vi "datataker_binary.vi"() -> ()   [LabVIEW 2012]
doc: "This example demonstrates how to acquire a single buffer of voltage measurements using a DAQmx device.\n\nFor instructions on how to connect your signals to the DAQ device, refer to your device documentation."
uses:
  <vilib>/userdefined/High Color/nirio_resource_hc.ctl
  <vilib>/Utility/error.llb/DialogType.ctl
  <vilib>/addons/h5labview2/file/H5Fmode.ctl
  <vilib>/DAQmx/write.llb/DAQmx Write (Analog 1D DBL 1Chan NSamp).vi
  <vilib>/DAQmx/read.llb/DAQmx Read (Analog 2D DBL NChan NSamp).vi
  <vilib>/addons/h5labview2/base/lib_path.vi
  <vilib>/DAQmx/read.llb/DAQmx Read (Analog 1D Wfm NChan NSamp).vi
  <vilib>/FPGAPlugInAG/PCIe-7841R/niLvFpga_Open_PCIe-7841R.vi
  <vilib>/DAQmx/create/channels.llb/DAQmx Create Channel (AI-Voltage-Basic).vi
  <vilib>/DAQmx/configure/timing.llb/DAQmx Timing (Sample Clock).vi
  <vilib>/DAQmx/configure/task.llb/DAQmx Configure Logging (TDMS).vi
  <vilib>/DAQmx/configure/trigger.llb/DAQmx Start Trigger (Digital Edge).vi
  <vilib>/DAQmx/configure/trigger.llb/DAQmx Start Trigger (Analog Edge).vi
  <vilib>/DAQmx/configure/trigger.llb/DAQmx Reference Trigger (Digital Edge).vi
  <vilib>/DAQmx/configure/trigger.llb/DAQmx Reference Trigger (Analog Edge).vi
  <vilib>/Utility/error.llb/Error Cluster From Error Code.vi
  <vilib>/rvi/errors/niLvFpgaAdjustHostInterfaceError.vi
  <vilib>/DAQmx/miscellaneous.llb/DAQmx Fill In Error Info.vi
  <vilib>/addons/h5labview2/base/H5Equery.vi
  Multiple Waveforms.vi
  <vilib>/Waveform/WDTFileIO.llb/Export Waveforms To Spreadsheet File (1D).vi
  <vilib>/DAQmx/create/channels.llb/DAQmx Create Channel (AO-Voltage-Basic).vi
  <vilib>/rvi/interface/nirviOpenFPGA/nirviOpenFPGA.xnode
  fpga/MultiChannelFeed_FPGATarget2_feedbackcooling(_T5hmXv3JUos.lvbitx
  <vilib>/rvi/interface/nirviReadWriteControl/nirviReadWriteControl.xnode
  <vilib>/addons/h5labview2/dataset/H5Dwrite.llb/H5Dwrite.xnode
  <vilib>/addons/h5labview2/attrib/H5Awrite.llb/H5Awrite.xnode
  <resource>/objmgr/daqmx.rc
  <vilib>/addons/h5labview2/file/H5F.lvlib
  <vilib>/addons/h5labview2/group/H5G.lvlib
  NiFpgaLv.dll
panel:
  in  "# Pulses":i32
  in  "Output channel (for flashing)":tag="Dev1/ao0"
  in  "Number of cyles\nbetween flashes":i32=100
  in  "Flash lamp?":bool
  out "error out":errorcluster
  in  "File base name":string="41Hz_250mV_1027Hz_1mVref"
  in  "Delay time between files(s)":dbl caption="Delay Time (s)"
  in  "Num files":i32=10000
  out "Array":dbl[](array[numeric])=[22.8, 23.9]
  in  "VISA Refnum in":refnum<visa-resource-name>="GPIB0::19::INSTR"
  in  "RIO Device":T1="RIO0::INSTR"
  in  "File type":string="Binary"
  in  "Directory path":path=path "D:/Data/20140529/Bead1/test"
  in  "Trigger Type":T2(tab)
  in  "Edge":i32(ring)=10280 items=["Rising"=10280, "Falling"=10171]
  in  "Digital Trigger Source":tag
  in  "Level (V)":dbl format="%0.2f"
  in  "Hysteresis (V)":dbl
  in  "Slope":i32(ring)=10280 items=["Rising"=10280, "Falling"=10171]
  in  "Analog Trigger Source":string="APFI0"
  in  "Digital Ref Trigger Source":tag
  in  "Edge":i32(ring)=10280 items=["Rising"=10280, "Falling"=10171]
  in  "Pre-Trigger Samples":u32
  in  "Analog Ref Trigger Source":string="APFI0"
  in  "Slope":i32(ring)=10280 items=["Rising"=10280, "Falling"=10171]
  in  "Level (V)":dbl format="%0.2f"
  in  "Pre-Trigger Samples":u32
  out "Waveform Graph":dbl[][](graph)
  in  "TDMS File Path":path
  in  "Number of Samples":i32=100000
  in  "Sample Rate":dbl=5000.0
  in  "Sample Clock Source":tag="OnboardClock"
  in  "Terminal Configuration":i32(ring)=-1 items=["default"=-1, "RSE"=10083, "NRSE"=10078, "Differential"=10106, "Pseudodifferential"=12529]
  in  "Max Voltage":dbl=5.0
  in  "Physical Channel":tag="Dev1/ai0:3"
  out "Actual Sample Rate":dbl=5000.0 format="%0.2f"
  in  "Logging Mode":i32(ring)=10231 items=["Off"=10231, "Log and Read"=15842]
  # "Channel Settings"
  # "Acquired Data"
  # "Timing Settings"
  # "Trigger Settings"
  # "Logging Settings"
  # "To configure and use a start trigger you must have the necessary tab selected above.  Not all hardware supports triggering--refer to your device documentation for more info."
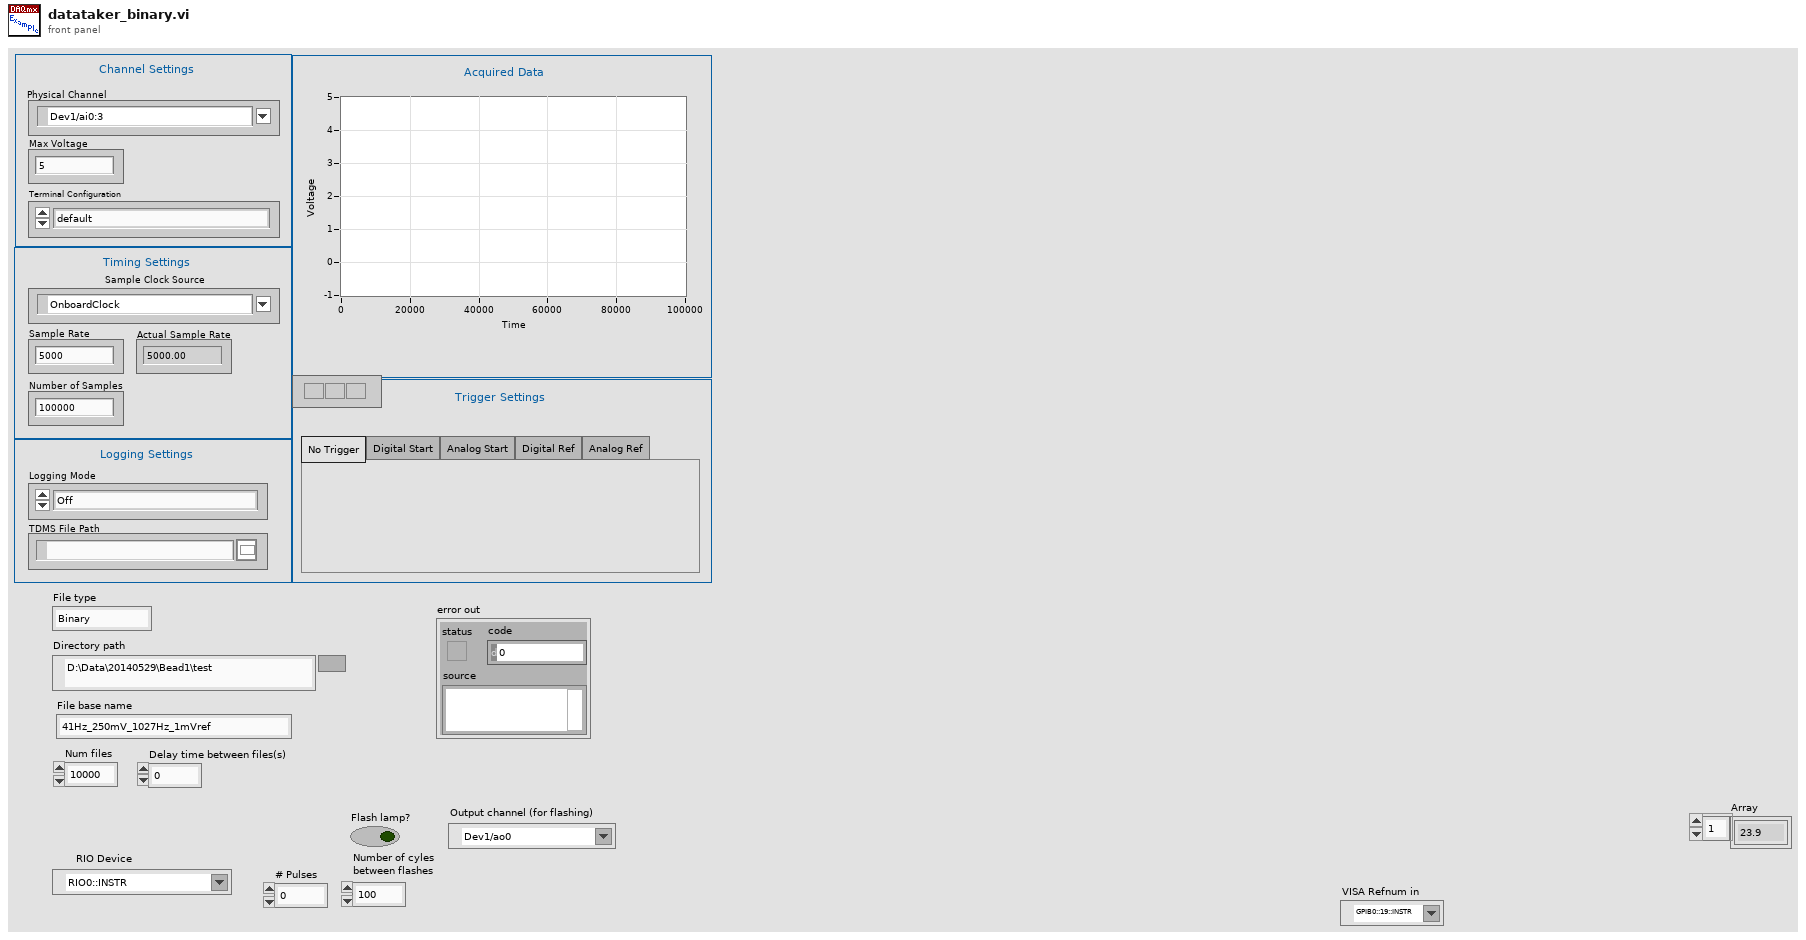
[diagram p1: front panel]
types:
  T1 = typedef "nirio_resource_hc.ctl" = tag
  T2 = enum32{"No Trigger", "Digital Start", "Analog Start", "Digital Ref", "Analog Ref"}
  T3 = typedef "H5F.lvlib/H5Fmode.ctl" = enum16{"read-only", "read-write", "overwrite", "create new", "open or create"}
  T4 = typedef "DialogType.ctl" = u16
  T5 = typedef "hid_t.ctl" = i32
  T6 = cluster{"pg 0":fxp<+/-,32,16>, "dg 0":fxp<+/-,32,16>, "pg 1":fxp<+/-,32,16>, "dg 1":fxp<+/-,32,16>, "pg 2":fxp<+/-,32,16>, "dg 2":fxp<+/-,32,16>, "Dc offset 0":fxp<+/-,32,16>, "Dc offset 1":fxp<+/-,32,16>, "Dc offset 2":fxp<+/-,32,16>}
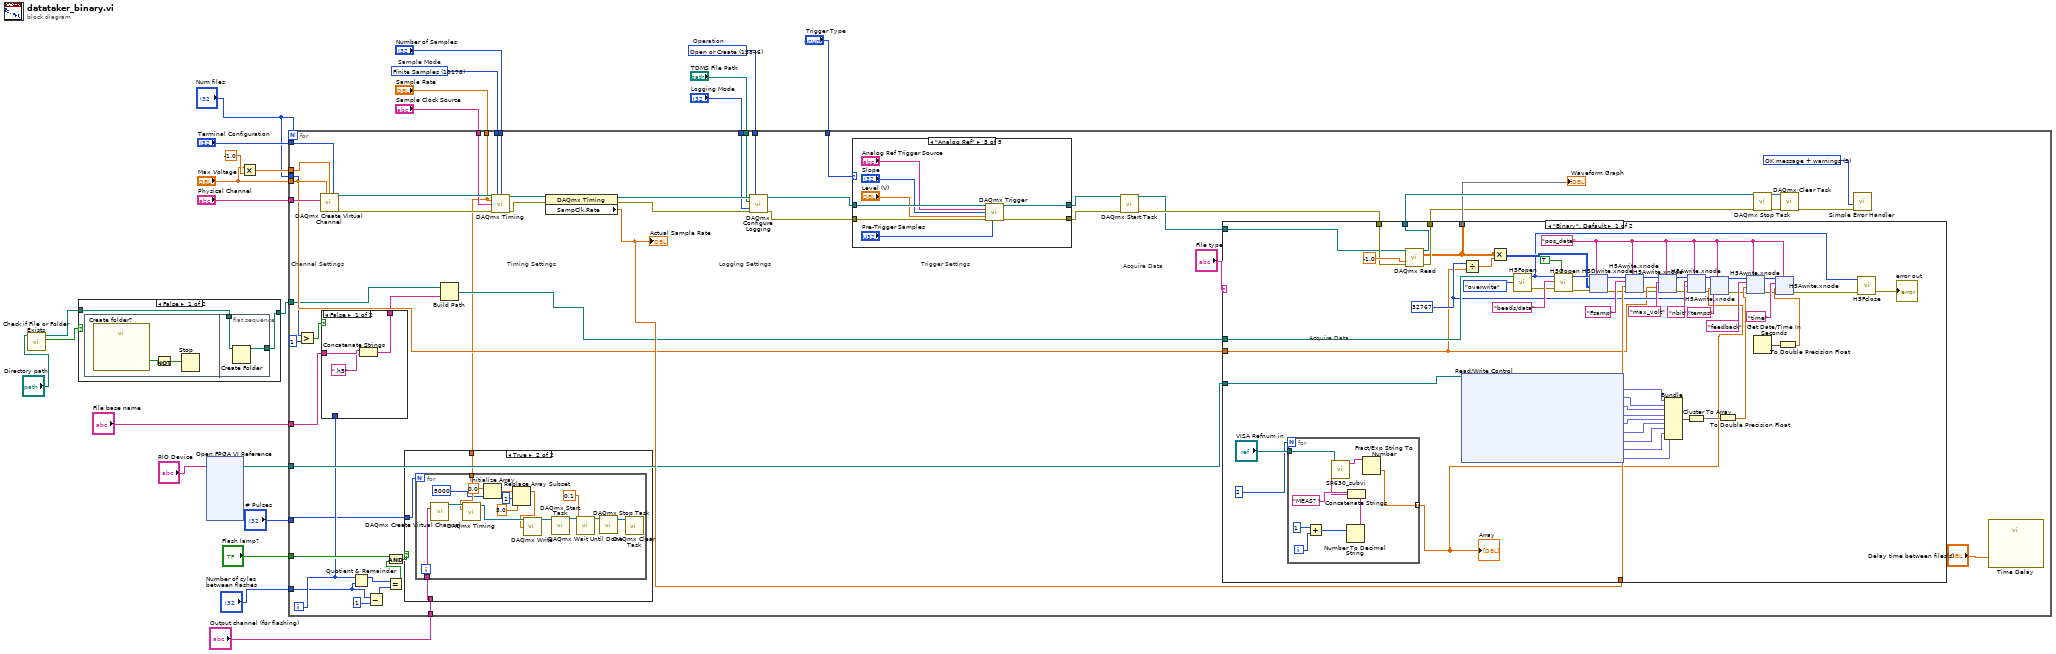
[diagram p0: block diagram]
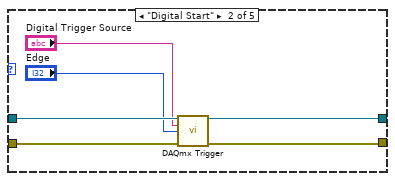
[diagram p5: hidden frame]
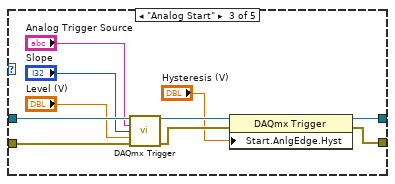
[diagram p6: hidden frame]
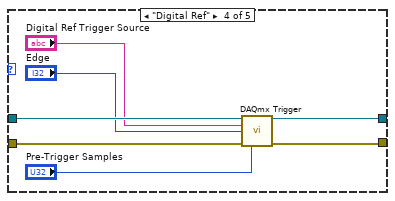
[diagram p7: hidden frame]
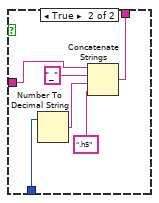
[diagram p8: hidden frame]
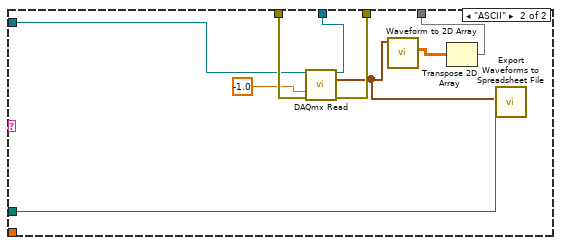
[diagram p9: hidden frame]
diagram:
  w24 = 15846 items=["Open"=10437, "Open or Create"=15846, "Create or Replace"=15847, "Create"=15848]  # Operation
  w25 = 10178 items=["Finite Samples"=10178, "Continuous Samples"=10123, "Hardware Timed Single Point"=12522]  # Sample Mode
  n1 = call <vilib>:"Check if File or Folder Exists.vi"("path"="Directory path") -> ("file or folder exists?"=w10:bool, "dup path"=w9:path)  [unwired: 8 in, 1 out]
  n2 = case shown="False" w10 {
    tunnel: w9 -> [w27 w32]
    tunnel: [w26 w32] -> w8
    frame False {
      n3 = flat-sequence {
        tunnel: w27 -> [w31]
        tunnel: [w30] -> w26
        frame #0 {
          n4 = call "Create folder?"() -> ("OK"=w29:bool)  [unwired: 18 in, 1 out]
          n5 = Not(x=w29) -> (.not. x?=w28:bool)
          n6 = Stop(stop? (T)=w28) -> ()
        }
        frame #1 {
          n7 = Create Folder(path (use dialog)=w31) -> (created path=w30:path)  [unwired: 2 in, 2 out]
        }
      }
    }
    frame True {
    }
  }
  n8 = xnode "Open FPGA VI Reference"("resource name"="RIO Device") -> ("FPGA VI Reference Out"=w12:refnum<k20>)  [unwired: 1 in, 1 out]
  n9 = Multiply(x="Max Voltage", y=-1.0) -> (x*y=w15:dbl)
  n10 = for {
    N: "Num files" -> [_]
    tunnel: w25 -> [w83]
    tunnel: w24 -> [w78]
    tunnel: "Logging Mode" -> [w76]
    tunnel: "Physical Channel" -> [w75]
    tunnel: "Terminal Configuration" -> [w74]
    tunnel: "Sample Clock Source" -> [w73]
    tunnel: "Sample Rate" -> [w35]
    tunnel: "TDMS File Path" -> [w72]
    tunnel: "Number of Samples" -> [w71]
    tunnel: w15 -> [w60]
    tunnel: "Max Voltage" -> [w59]
    tunnel: w12 -> [w58]
    tunnel: w8 -> [w56]
    tunnel: "Num files" -> [w55]
    tunnel: "File base name" -> [w51]
    tunnel: "Trigger Type" -> [w45]
    tunnel: "Flash lamp?" -> [w44]
    tunnel: "Number of cyles\nbetween flashes" -> [w34]
    tunnel: "Output channel (for flashing)" -> [w37]
    tunnel: "# Pulses" -> [w33]
    i -> [w41]
    w68 = T4 3 items=["no dialog", "OK message", "continue or stop message", "OK message + warnings", "continue/stop + warnings"] ("type of dialog (OK msg:1)")
    # "Acquire Data"
    # "Acquire Data"
    # "Trigger Settings"
    # "Timing Settings"
    # "Channel Settings"
    # "Logging Settings"
    n11 = Greater?(x=w55, y=1) -> (0:w53:bool)
    n12 = call-poly <vilib>:"DAQmx Create Virtual Channel.vi"("maximum value"=w59, "minimum value"=w60, "input terminal configuration"=w74, "physical channels"=w75) -> ("task out"=w81:refnum<k21>, "error out"=w82:errorcluster)  [unwired: 10 in]
    n13 = case shown="False" w53 {
      tunnel: w51 -> [w138 w144]
      tunnel: w41 -> [_ w141]
      tunnel: [w136 w139] -> w50
      frame False {
        n14 = Concatenate Strings(w138, ".h5" ("string")) -> (w136:string)
      }
      frame True {
        n15 = Number To Decimal String(number=w141) -> (decimal integer string=w142:string)  [unwired: 1 in]
        n16 = Concatenate Strings(w144, "_" ("string"), w142, ".h5" ("string")) -> (w139:string)
      }
    }
    n17 = Quotient & Remainder(x=w41, y=w34) -> (x-y*floor(x/y)=w42:i32)  [unwired: 1 out]
    n18 = Subtract(x=w34, y=1) -> (x-y=w39:i32)
    n19 = Equal?(x=w42, y=w39) -> (x = y?=w38:bool)
    n20 = And(x=w44, y=w38) -> (x .and. y?=w43:bool)
    n21 = case shown="True" w43 {
      tunnel: w37 -> [_ w87]
      tunnel: w35 -> [_ w86]
      tunnel: w33 -> [_ w85]
      frame False {
      }
      frame True {
        n22 = for {
          N: w85 -> [_]
          tunnel: w87 -> [w102]
          tunnel: w86 -> [w99]
          n23 = call-poly <vilib>:"DAQmx Create Virtual Channel.vi"("physical channels"=w102) -> ("task out"=w100:refnum<k21>)  [unwired: 13 in, 1 out]
          n24 = call-poly <vilib>:"DAQmx Timing.vi"("task/channels in"=w100, "rate"=w99) -> ("task out"=w93:refnum<k21>)  [unwired: 12 in, 1 out]
          n25 = Initialize Array(0.0 ("element"), 5000 ("dimension size")) -> (w96:dbl[])
          n26 = Replace Array Subset(array=w96, new element=5.0 ("new element/subarray"), index=1) -> (w92:dbl[])
          n27 = call-poly <vilib>:"DAQmx Write.vi"("task/channels in"=w93, "data"=w92) -> ("task out"=w91:refnum<k21>)  [unwired: 11 in, 2 out]
          n28 = call <vilib>:"DAQmx Start Task.vi"("task/channels in"=w91) -> ("task out"=w90:refnum<k21>)  [unwired: 13 in, 1 out]
          n29 = call <vilib>:"DAQmx Wait Until Done.vi"("task/channels in"=w90, "timeout (sec)"=0.1) -> ("task out"=w89:refnum<k21>)  [unwired: 12 in, 1 out]
          n30 = call <vilib>:"DAQmx Stop Task.vi"("task/channels in"=w89) -> ("task out"=w101:refnum<k21>)  [unwired: 13 in, 1 out]
          n31 = call <vilib>:"DAQmx Clear Task.vi"("task in"=w101) -> ()  [unwired: 14 in, 1 out]
        }
      }
    }
    n32 = Build Path(base path=w56, name or relative path=w50) -> (appended path=w52:path)
    n33 = call-poly <vilib>:"DAQmx Timing.vi"("task/channels in"=w81, "sample mode"=w83, "samples per channel"=w71, "rate"=w35, "source"=w73, "error in"=w82) -> ("task out"=w36:refnum<k21>, "error out"=w84:errorcluster)  [unwired: 8 in]
    n34 = property class="DAQmx Timing"(reference=w36, error in=w84) -> (reference out=w80:refnum<k21>, error out=w79:errorcluster, "SampClk.Rate"=w66:dbl)
    "Actual Sample Rate" <- w66
    n35 = call-poly <vilib>:"DAQmx Configure Logging.vi"("task/channels in"=w80, "operation"=w78, "file path"=w72, "logging mode"=w76, "error in"=w79) -> ("task out"=w49:refnum<k21>, "error out"=w48:errorcluster)  [unwired: 9 in]
    n36 = case shown="\"Analog Ref\"" w45 {
      tunnel: w49 -> [w104 w110 w120 w127 w135]
      tunnel: w48 -> [w103 w109 w119 w126 w134]
      tunnel: [w104 w108 w117 w125 w129] -> w46
      tunnel: [w103 w107 w116 w124 w130] -> w47
      frame "No Trigger", Default {
      }
      frame "Digital Start" {
        n37 = call-poly <vilib>:"DAQmx Trigger.vi"("task/channels in"=w110, "source"="Digital Trigger Source", "edge"="Edge", "error in"=w109) -> ("task out"=w108:refnum<k21>, "error out"=w107:errorcluster)  [unwired: 10 in]
      }
      frame "Analog Start" {
        n38 = call-poly <vilib>:"DAQmx Trigger.vi"("task/channels in"=w120, "source"="Analog Trigger Source", "slope"="Slope", "level"="Level (V)", "error in"=w119) -> ("task out"=w115:refnum<k21>, "error out"=w114:errorcluster)  [unwired: 9 in]
        n39 = property class="DAQmx Trigger"(reference=w115, error in=w114, "Start.AnlgEdge.Hyst"="Hysteresis (V)") -> (reference out=w117:refnum<k21>, error out=w116:errorcluster)
      }
      frame "Digital Ref" {
        n40 = call-poly <vilib>:"DAQmx Trigger.vi"("task/channels in"=w127, "source"="Digital Ref Trigger Source", "edge"="Edge", "error in"=w126, "pretrigger samples per channel"="Pre-Trigger Samples") -> ("task out"=w125:refnum<k21>, "error out"=w124:errorcluster)  [unwired: 9 in]
      }
      frame "Analog Ref" {
        n41 = call-poly <vilib>:"DAQmx Trigger.vi"("task/channels in"=w135, "source"="Analog Ref Trigger Source", "slope"="Slope", "level"="Level (V)", "error in"=w134, "pretrigger samples per channel"="Pre-Trigger Samples") -> ("task out"=w129:refnum<k21>, "error out"=w130:errorcluster)  [unwired: 8 in]
      }
    }
    n42 = call <vilib>:"DAQmx Start Task.vi"("task/channels in"=w46, "error in"=w47) -> ("task out"=w64:refnum<k21>, "error out"=w65:errorcluster)  [unwired: 12 in]
    n43 = case shown="\"Binary\", Default" "File type" {
      tunnel: w52 -> [w202 w346]
      tunnel: w66 -> [w195 _]
      tunnel: w65 -> [w193 w345]
      tunnel: w64 -> [w190 w344]
      tunnel: [w191 w342] -> w63
      tunnel: [w185 w338] -> w62
      tunnel: [w192 w341] -> w61
      tunnel: w59 -> [w182 _]
      tunnel: w58 -> [w158 _]
      frame "Binary", Default {
        w183 = i16 32767 ("y")
        w163 = "pos_data" ("dataset name")
        n44 = for {
          N: 2 ("dimension size") -> [_]
          tunnel: "VISA Refnum in" -> [w211]
          tunnel: [w209] -> w159 mode=indexing
          i -> [w208]
          n45 = Add(x=1, y=w208) -> (x+y=w206:i32)
          n46 = Number To Decimal String(number=w206) -> (decimal integer string=w205:string)  [unwired: 1 in]
          n47 = Concatenate Strings("MEAS? " ("Write Buffer"), w205) -> (w203:string)
          n48 = call "SR630_subvi.vi"("Write Buffer"=w203, "VISA Refnum in"=w211) -> ("read buffer"=w210:string)  [unwired: 9 in]
          n49 = Fract/Exp String To Number(string=w210) -> (number=w209:dbl)  [unwired: 3 in, 1 out]
        }
        "Array" <- w159
        n50 = call-poly <vilib>:"DAQmx Read.vi"("task/channels in"=w190, "timeout"=-1.0, "error in"=w193) -> ("task out"=w191:refnum<k21>, "data"=w185:dbl[][], "error out"=w192:errorcluster)  [unwired: 10 in]
        n51 = xnode "Read/Write Control"("FPGA VI Reference In"=w158) -> ("pg 0"=w175:fxp<+/-,32,16>, "dg 0"=w174:fxp<+/-,32,16>, "pg 1"=w173:fxp<+/-,32,16>, "dg 1"=w172:fxp<+/-,32,16>, "pg 2"=w171:fxp<+/-,32,16>, "dg 2"=w170:fxp<+/-,32,16>, "Dc offset 0"=w169:fxp<+/-,32,16>, "Dc offset 1"=w168:fxp<+/-,32,16>, "Dc offset 2"=w167:fxp<+/-,32,16>)  [unwired: 1 in, 2 out]
        n52 = Divide(x=w183, y=w182) -> (x/y=w184:dbl)
        n53 = Multiply(x=w185, y=w184) -> (x*y=w181:i16[][])
        n54 = call <vilib>:"H5Fopen.vi"("mode (read-only)"=H5Fmode."overwrite", "path"=w202) -> ("error out"=w155:errorcluster, "ref out"=w145:T5)  [unwired: 2 in]
        n55 = call <vilib>:"H5Gopen.vi"("create? (F)"=TRUE, "error in (no error)"=w155, "name"="beads/data", "ref in"=w145) -> ("error out"=w154:errorcluster, "group out"=w198:T5)  [unwired: 3 in]
        n56 = xnode "H5Dwrite.xnode"("dataset name"=w163, "error in (no error)"=w154, "data"=w181, "ref in"=w198) -> ("error out"=w153:errorcluster, "ref out"=w197:i32)  [unwired: 3 in, 1 out]
        n57 = xnode "H5Awrite.xnode"("object name"=w163, "error in (no error)"=w153, "data"=w195, "attrib name"="Fsamp", "ref in"=w197) -> ("error out"=w152:errorcluster, "ref out"=w189:i32)  [unwired: 2 in, 1 out]
        n58 = xnode "H5Awrite.xnode"("object name"=w163, "error in (no error)"=w152, "data"=w182, "attrib name"="max_volt", "ref in"=w189) -> ("error out"=w151:errorcluster, "ref out"=w187:i32)  [unwired: 2 in, 1 out]
        n59 = Bundle("pg 0"=w175, "dg 0"=w174, "pg 1"=w173, "dg 1"=w172, "pg 2"=w171, "dg 2"=w170, "Dc offset 0"=w169, "Dc offset 1"=w168, "Dc offset 2"=w167) -> (w176:T6)  [unwired: 1 in]
        n60 = xnode "H5Awrite.xnode"("object name"=w163, "error in (no error)"=w151, "data"=w183, "attrib name"="nbit", "ref in"=w187) -> ("error out"=w150:errorcluster, "ref out"=w179:i32)  [unwired: 2 in, 1 out]
        n61 = Cluster To Array(cluster=w176) -> (array=w166:fxp<+/-,32,16>[])
        n62 = xnode "H5Awrite.xnode"("object name"=w163, "error in (no error)"=w150, "data"=w159, "attrib name"="temps", "ref in"=w179) -> ("error out"=w149:errorcluster, "ref out"=w178:i32)  [unwired: 2 in, 1 out]
        n63 = To Double Precision Float(number=w166) -> (double precision float=w165:dbl[])
        n64 = xnode "H5Awrite.xnode"("object name"=w163, "error in (no error)"=w149, "data"=w165, "attrib name"="feedback", "ref in"=w178) -> ("error out"=w148:errorcluster, "ref out"=w162:i32)  [unwired: 2 in, 1 out]
        n65 = Get Date/Time In Seconds() -> (seconds since 1Jan1904=w157:timestamp)
        n66 = To Double Precision Float(number=w157) -> (double precision float=w156:dbl)
        n67 = xnode "H5Awrite.xnode"("object name"=w163, "error in (no error)"=w148, "data"=w156, "attrib name"="time", "ref in"=w162) -> ("error out"=w146:errorcluster)  [unwired: 2 in, 2 out]
        n68 = call <vilib>:"H5Fclose.vi"("error in (no error)"=w146, "ref"=w145) -> ("error out"=→"error out":errorcluster)  [unwired: 3 in]
      }
      frame "ASCII" {
        n69 = call-poly <vilib>:"DAQmx Read.vi"("task/channels in"=w344, "timeout"=-1.0, "error in"=w345) -> ("task out"=w342:refnum<k21>, "data"=w340:waveform(dbl)[], "error out"=w341:errorcluster)  [unwired: 10 in]
        n70 = call-poly "Waveform to 2D Array.vi"("Multiple Waveforms"=w340) -> ("2D Array"=w339:dbl[][])  [unwired: 9 in, 1 out]
        n71 = Transpose 2D Array(2D array=w339) -> (transposed array=w338:dbl[][])
        n72 = call-poly <vilib>:"Export Waveforms to Spreadsheet File.vi"("waveforms"=w340, "file path (dialog if empty)"=w346) -> ()  [unwired: 8 in, 2 out]
      }
    }
    "Waveform Graph" <- w62
    n73 = call <vilib>:"DAQmx Stop Task.vi"("task/channels in"=w63, "error in"=w61) -> ("task out"=w70:refnum<k21>, "error out"=w69:errorcluster)  [unwired: 12 in]
    n74 = call <vilib>:"DAQmx Clear Task.vi"("task in"=w70, "error in"=w69) -> ("error out"=w77:errorcluster)  [unwired: 13 in]
    n75 = call <vilib>:"Simple Error Handler.vi"("type of dialog (OK msg:1)"=w68, "error in (no error)"=w77) -> ()  [unwired: 3 in, 5 out]
    n76 = call "Time Delay"("Delay Time (s)"="Delay time between files(s)") -> ()  [unwired: 10 in, 1 out]
  }
